vi "FpgaLink_Error_Handler.vi"(8 "error in (no error)":errorcluster, 10 "error string":string, 11 "error code":i32) -> (0 "error out":errorcluster)   [LabVIEW 2011]
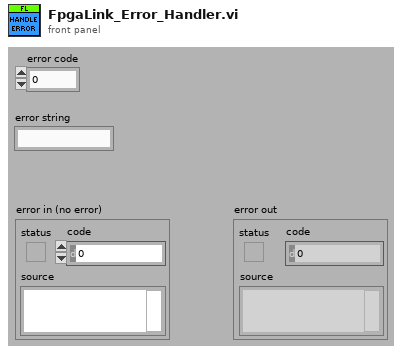
[diagram p1: front panel]
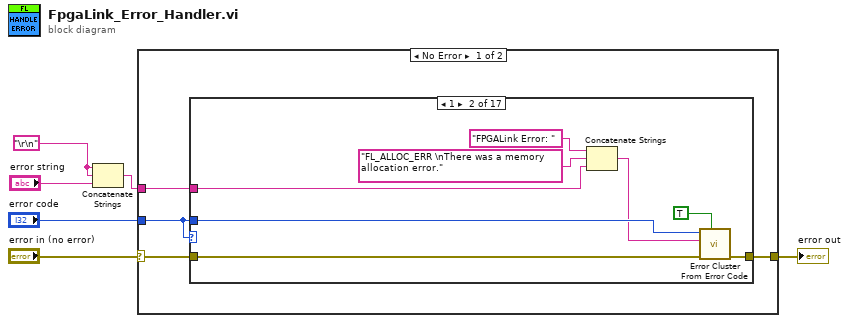
[diagram p0: block diagram]
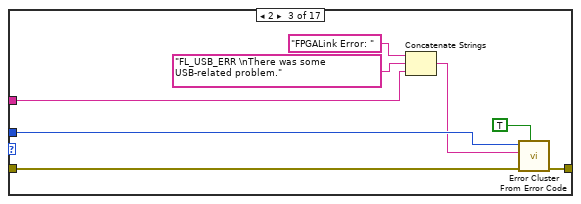
[diagram p3: hidden frame]
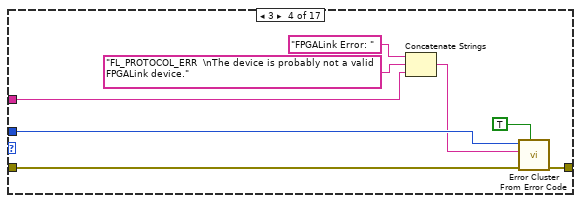
[diagram p4: hidden frame]
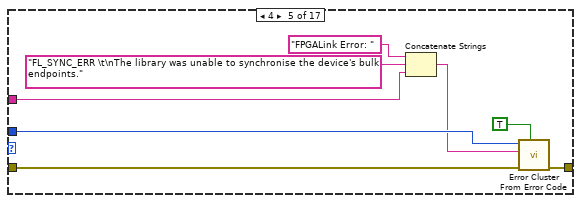
[diagram p5: hidden frame]
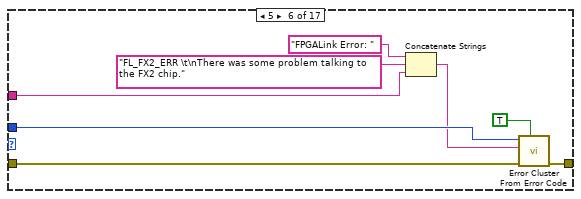
[diagram p6: hidden frame]
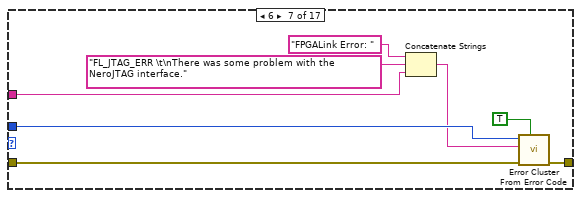
[diagram p7: hidden frame]
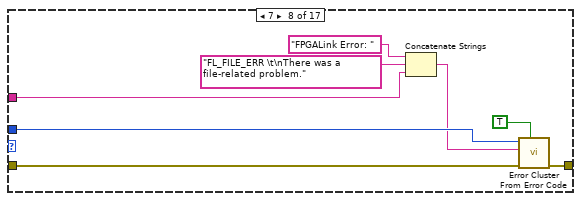
[diagram p8: hidden frame]
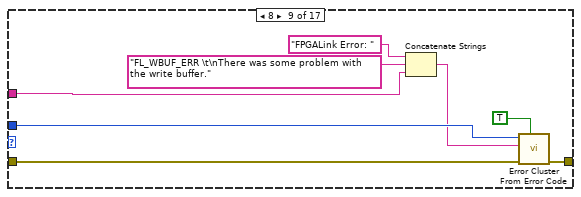
[diagram p9: hidden frame]
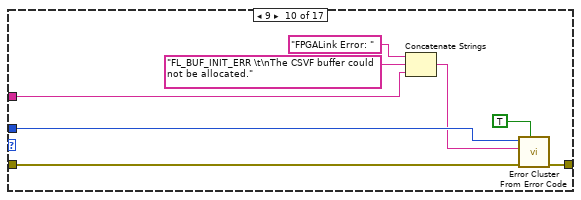
[diagram p10: hidden frame]
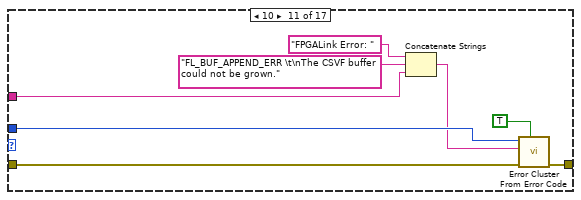
[diagram p11: hidden frame]
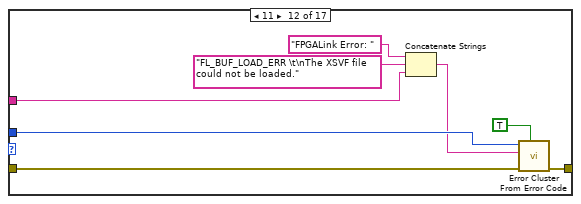
[diagram p12: hidden frame]
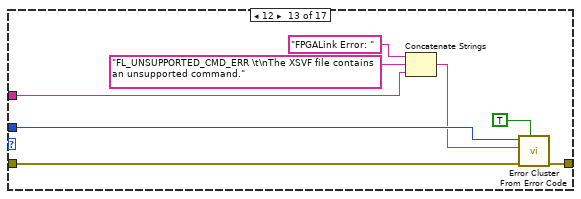
[diagram p13: hidden frame]
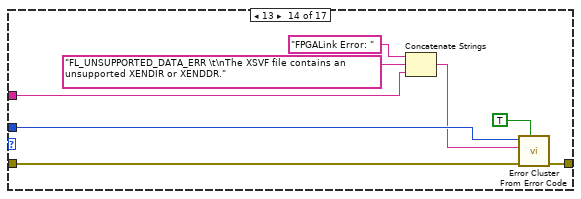
[diagram p14: hidden frame]
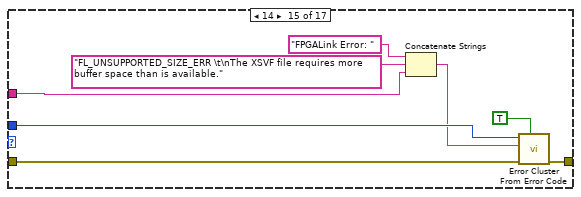
[diagram p15: hidden frame]
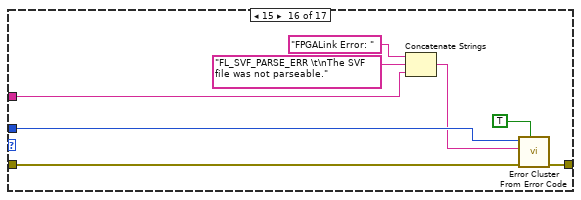
[diagram p16: hidden frame]
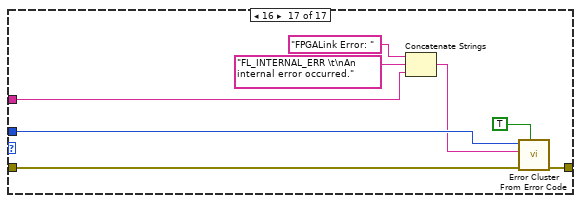
[diagram p17: hidden frame]
diagram:
  w1 = "\r\n"
  n1 = Concatenate Strings(w1, w1, "error string") -> (w3:string)
  n2 = case shown="No Error" "error in (no error)" {
    selector: "error in (no error)" -> [w10 w140]
    tunnel: [w9 w140] -> w5
    tunnel: "error code" -> [w8 _]
    tunnel: w3 -> [w7 _]
    frame No Error {
      n3 = case shown="1" w8 {
        tunnel: w10 -> [w11 w19 w27 w35 w43 w51 w59 w67 w75 w83 w91 w99 w107 w115 w123 w131 w139]
        tunnel: w8 -> [_ w17 w25 w33 w41 w49 w57 w65 w73 w81 w89 w97 w105 w113 w121 w129 w137]
        tunnel: [w11 w18 w26 w34 w42 w50 w58 w66 w74 w82 w90 w98 w106 w114 w122 w130 w138] -> w9
        tunnel: w7 -> [_ w12 w20 w28 w36 w44 w52 w60 w68 w76 w84 w92 w100 w108 w116 w124 w132]
        frame 0, Default {
        }
        frame 1 {
          n4 = Concatenate Strings("FPGALink Error: ", "FL_ALLOC_ERR \nThere was a memory allocation error." ("string"), w12) -> (w13:string)
          n5 = call <vilib>:"Error Cluster From Error Code.vi"("show call chain? (False)"=TRUE, "error in (no error)"=w19, "error message (\"\")"=w13, "error code (0)"=w17) -> ("error out"=w18:errorcluster)  [unwired: 5 in]
        }
        frame 2 {
          n6 = Concatenate Strings("FPGALink Error: ", "FL_USB_ERR \nThere was some USB-related problem." ("string"), w20) -> (w21:string)
          n7 = call <vilib>:"Error Cluster From Error Code.vi"("show call chain? (False)"=TRUE, "error in (no error)"=w27, "error message (\"\")"=w21, "error code (0)"=w25) -> ("error out"=w26:errorcluster)  [unwired: 5 in]
        }
        frame 3 {
          n8 = Concatenate Strings("FPGALink Error: ", "FL_PROTOCOL_ERR  \nThe device is probably not a valid FPGALink device." ("string"), w28) -> (w29:string)
          n9 = call <vilib>:"Error Cluster From Error Code.vi"("show call chain? (False)"=TRUE, "error in (no error)"=w35, "error message (\"\")"=w29, "error code (0)"=w33) -> ("error out"=w34:errorcluster)  [unwired: 5 in]
        }
        frame 4 {
          n10 = Concatenate Strings("FPGALink Error: ", "FL_SYNC_ERR \t\nThe library was unable to synchronise the device's bulk endpoints." ("string"), w36) -> (w37:string)
          n11 = call <vilib>:"Error Cluster From Error Code.vi"("show call chain? (False)"=TRUE, "error in (no error)"=w43, "error message (\"\")"=w37, "error code (0)"=w41) -> ("error out"=w42:errorcluster)  [unwired: 5 in]
        }
        frame 5 {
          n12 = Concatenate Strings("FPGALink Error: ", "FL_FX2_ERR \t\nThere was some problem talking to the FX2 chip." ("string"), w44) -> (w45:string)
          n13 = call <vilib>:"Error Cluster From Error Code.vi"("show call chain? (False)"=TRUE, "error in (no error)"=w51, "error message (\"\")"=w45, "error code (0)"=w49) -> ("error out"=w50:errorcluster)  [unwired: 5 in]
        }
        frame 6 {
          n14 = Concatenate Strings("FPGALink Error: ", "FL_JTAG_ERR \t\nThere was some problem with the NeroJTAG interface." ("string"), w52) -> (w53:string)
          n15 = call <vilib>:"Error Cluster From Error Code.vi"("show call chain? (False)"=TRUE, "error in (no error)"=w59, "error message (\"\")"=w53, "error code (0)"=w57) -> ("error out"=w58:errorcluster)  [unwired: 5 in]
        }
        frame 7 {
          n16 = Concatenate Strings("FPGALink Error: ", "FL_FILE_ERR \t\nThere was a file-related problem." ("string"), w60) -> (w61:string)
          n17 = call <vilib>:"Error Cluster From Error Code.vi"("show call chain? (False)"=TRUE, "error in (no error)"=w67, "error message (\"\")"=w61, "error code (0)"=w65) -> ("error out"=w66:errorcluster)  [unwired: 5 in]
        }
        frame 8 {
          n18 = Concatenate Strings("FPGALink Error: ", "FL_WBUF_ERR \t\nThere was some problem with the write buffer." ("string"), w68) -> (w69:string)
          n19 = call <vilib>:"Error Cluster From Error Code.vi"("show call chain? (False)"=TRUE, "error in (no error)"=w75, "error message (\"\")"=w69, "error code (0)"=w73) -> ("error out"=w74:errorcluster)  [unwired: 5 in]
        }
        frame 9 {
          n20 = Concatenate Strings("FPGALink Error: ", "FL_BUF_INIT_ERR \t\nThe CSVF buffer could not be allocated." ("string"), w76) -> (w77:string)
          n21 = call <vilib>:"Error Cluster From Error Code.vi"("show call chain? (False)"=TRUE, "error in (no error)"=w83, "error message (\"\")"=w77, "error code (0)"=w81) -> ("error out"=w82:errorcluster)  [unwired: 5 in]
        }
        frame 10 {
          n22 = Concatenate Strings("FPGALink Error: ", "FL_BUF_APPEND_ERR \t\nThe CSVF buffer could not be grown." ("string"), w84) -> (w85:string)
          n23 = call <vilib>:"Error Cluster From Error Code.vi"("show call chain? (False)"=TRUE, "error in (no error)"=w91, "error message (\"\")"=w85, "error code (0)"=w89) -> ("error out"=w90:errorcluster)  [unwired: 5 in]
        }
        frame 11 {
          n24 = Concatenate Strings("FPGALink Error: ", "FL_BUF_LOAD_ERR \t\nThe XSVF file could not be loaded." ("string"), w92) -> (w93:string)
          n25 = call <vilib>:"Error Cluster From Error Code.vi"("show call chain? (False)"=TRUE, "error in (no error)"=w99, "error message (\"\")"=w93, "error code (0)"=w97) -> ("error out"=w98:errorcluster)  [unwired: 5 in]
        }
        frame 12 {
          n26 = Concatenate Strings("FPGALink Error: ", "FL_UNSUPPORTED_CMD_ERR \t\nThe XSVF file contains an unsupported command." ("string"), w100) -> (w101:string)
          n27 = call <vilib>:"Error Cluster From Error Code.vi"("show call chain? (False)"=TRUE, "error in (no error)"=w107, "error message (\"\")"=w101, "error code (0)"=w105) -> ("error out"=w106:errorcluster)  [unwired: 5 in]
        }
        frame 13 {
          n28 = Concatenate Strings("FPGALink Error: ", "FL_UNSUPPORTED_DATA_ERR \t\nThe XSVF file contains an unsupported XENDIR or XENDDR." ("string"), w108) -> (w109:string)
          n29 = call <vilib>:"Error Cluster From Error Code.vi"("show call chain? (False)"=TRUE, "error in (no error)"=w115, "error message (\"\")"=w109, "error code (0)"=w113) -> ("error out"=w114:errorcluster)  [unwired: 5 in]
        }
        frame 14 {
          n30 = Concatenate Strings("FPGALink Error: ", "FL_UNSUPPORTED_SIZE_ERR \t\nThe XSVF file requires more buffer space than is available." ("string"), w116) -> (w117:string)
          n31 = call <vilib>:"Error Cluster From Error Code.vi"("show call chain? (False)"=TRUE, "error in (no error)"=w123, "error message (\"\")"=w117, "error code (0)"=w121) -> ("error out"=w122:errorcluster)  [unwired: 5 in]
        }
        frame 15 {
          n32 = Concatenate Strings("FPGALink Error: ", "FL_SVF_PARSE_ERR \t\nThe SVF file was not parseable." ("string"), w124) -> (w125:string)
          n33 = call <vilib>:"Error Cluster From Error Code.vi"("show call chain? (False)"=TRUE, "error in (no error)"=w131, "error message (\"\")"=w125, "error code (0)"=w129) -> ("error out"=w130:errorcluster)  [unwired: 5 in]
        }
        frame 16 {
          n34 = Concatenate Strings("FPGALink Error: ", "FL_INTERNAL_ERR \t\nAn internal error occurred." ("string"), w132) -> (w133:string)
          n35 = call <vilib>:"Error Cluster From Error Code.vi"("show call chain? (False)"=TRUE, "error in (no error)"=w139, "error message (\"\")"=w133, "error code (0)"=w137) -> ("error out"=w138:errorcluster)  [unwired: 5 in]
        }
      }
    }
    frame Error {
    }
  }
  "error out" <- w5
